vi "Initialize Panel.vi"(8 "error in":errorcluster, 9 "MHL Configuration":T5, 10 "MHL References":T4, 11 "MHL UI Data in":T1) -> (0 "error out":errorcluster, 2 "MHL Data out":T3, 3 "MHL UI Data out":T1)   [LabVIEW 2015]
uses:
  controls/MHL References.ctl
  controls/MHL Configuration.ctl
  controls/MHL UI Data.ctl
  controls/MHL Status.ctl
  controls/MHL Data.ctl
  Boiler System Globals.vi
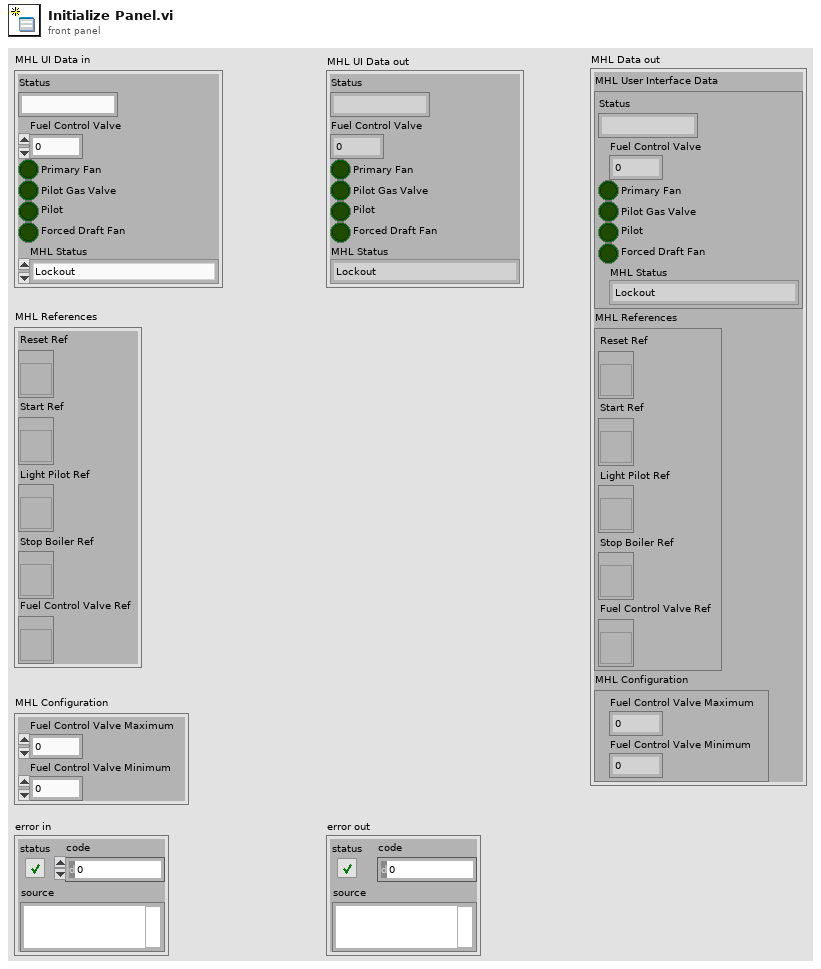
[diagram p1: front panel]
types:
  T1 = typedef "MHL UI Data.ctl" = cluster{"Status":string, "Fuel Control Valve":u32, "Primary Fan":bool, "Pilot Gas Valve":bool, "Pilot":bool, "Forced Draft Fan":bool, "MHL Status":T2}
  T2 = typedef "MHL Status.ctl" = enum16{"Lockout", "Ready", "Pre-Purge", "Pre-Purge Complete", "Pilot On", "Boiler Running", "Shutdown", "Purge"}
  T3 = typedef "MHL Data.ctl" = cluster{"MHL User Interface Data":T1, "MHL References":T4, "MHL Configuration":T5}
  T4 = typedef "MHL References.ctl" = cluster{"Reset Ref":refnum<vi>, "Start Ref":refnum<vi>, "Light Pilot Ref":refnum<vi>, "Stop Boiler Ref":refnum<vi>, "Fuel Control Valve Ref":refnum<vi>}
  T5 = typedef "MHL Configuration.ctl" = cluster{"Fuel Control Valve Maximum":dbl, "Fuel Control Valve Minimum":dbl}
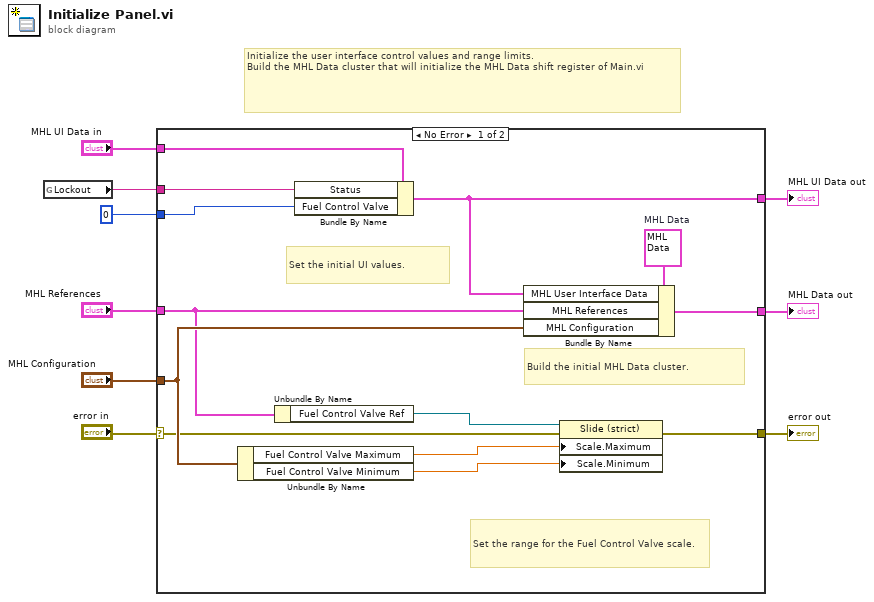
[diagram p0: block diagram]
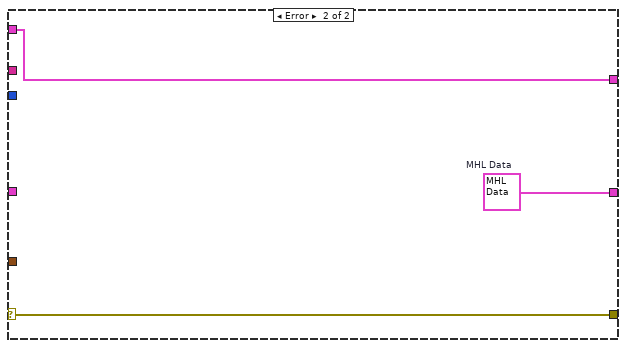
[diagram p2: hidden frame]
diagram:
  # "Initialize the user interface control values and range limits.\nBuild the MHL Data cluster that will initialize the MHL Data shift register of Main.vi"
  n1 = global read "Boiler System Globals.vi" "Lockout"() -> (w8:string)
  n2 = case shown="No Error" "error in" {
    selector: "error in" -> [w11 w25]
    tunnel: u32 0 ("Fuel Control Valve") -> [w19 _]
    tunnel: w8 -> [w18 _]
    tunnel: "MHL Configuration" -> [w16 _]
    tunnel: "MHL References" -> [w15 _]
    tunnel: "MHL UI Data in" -> [w14 w23]
    tunnel: [w13 w24] -> w4
    tunnel: [w12 w25] -> w3
    tunnel: [w10 w23] -> w1
    frame No Error {
      w17 = T3 {"MHL User Interface Data"={"Status"="", "Fuel Control Valve"=0, "Primary Fan"=FALSE, "Pilot Gas Valve"=FALSE, "Pilot"=FALSE, "Forced Draft Fan"=FALSE, "MHL Status"=enum."Lockout"}, "MHL References"={"Reset Ref"=refnum, "Start Ref"=refnum, "Light Pilot Ref"=refnum, "Stop Boiler Ref"=refnum, "Fuel Control Valve Ref"=refnum}, "MHL Configuration"={"Fuel Control Valve Maximum"=0.0, "Fuel Control Valve Minimum"=0.0}}  # MHL Data
      # "Build the initial MHL Data cluster."
      # "Set the range for the Fuel Control Valve scale."
      # "Set the initial UI values."
      n3 = Unbundle By Name(w16) -> ("Fuel Control Valve Maximum"=w21:dbl, "Fuel Control Valve Minimum"=w20:dbl)
      n4 = Unbundle By Name(w15) -> ("Fuel Control Valve Ref"=w22:refnum<vi>)
      n5 = Bundle By Name(cluster=w14, "Status"=w18, "Fuel Control Valve"=w19) -> (w10:T1)
      n6 = Bundle By Name(cluster=w17, "MHL User Interface Data"=w10, "MHL References"=w15, "MHL Configuration"=w16) -> (w13:T3)
      n7 = property class="Slide (strict)"(reference=w22, error in=w11, "Scale.Maximum"=w21, "Scale.Minimum"=w20) -> (error out=w12:errorcluster)  [unwired: 1 out]
    }
    frame Error {
      w24 = T3 {"MHL User Interface Data"={"Status"="", "Fuel Control Valve"=0, "Primary Fan"=FALSE, "Pilot Gas Valve"=FALSE, "Pilot"=FALSE, "Forced Draft Fan"=FALSE, "MHL Status"=enum."Lockout"}, "MHL References"={"Reset Ref"=refnum, "Start Ref"=refnum, "Light Pilot Ref"=refnum, "Stop Boiler Ref"=refnum, "Fuel Control Valve Ref"=refnum}, "MHL Configuration"={"Fuel Control Valve Maximum"=0.0, "Fuel Control Valve Minimum"=0.0}}  # MHL Data
    }
  }
  "MHL Data out" <- w4
  "error out" <- w3
  "MHL UI Data out" <- w1
